vi "CRYSave DataView GUI Info.vi"(11 "DataView Index":i32) -> (3 "DataView GUI Info":T1)   [LabVIEW 2013]
uses:
  Control/Graph Main Info Cluster.ctl
  Control/SplitterBar.ctl
  CRYNew View Global.vi
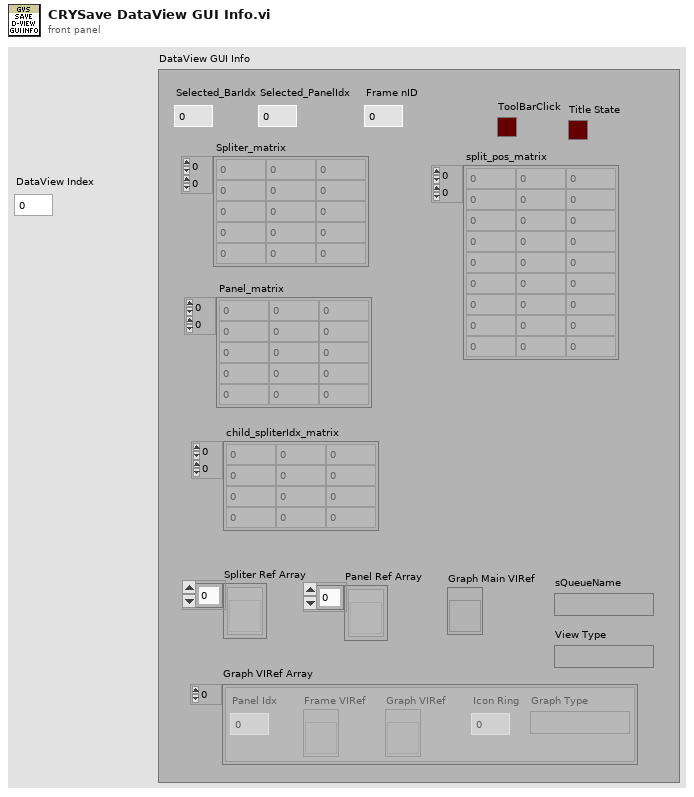
[diagram p1: front panel]
types:
  T1 = typedef "Graph Main Info Cluster.ctl" = cluster{"Selected_BarIdx":i32, "Selected_PanelIdx":i32, "Graph Main VIRef":refnum<vi>, "ToolBarClick":bool, "Spliter Ref Array":refnum<vi>[], "Panel Ref Array":refnum<vi>[], "Spliter_matrix":i32[][], "Panel_matrix":i32[][], "child_spliterIdx_matrix":i32[][], "split_pos_matrix":i32[][], "Title State":bool, "sQueueName":string, "Frame nID":i32, "Graph VIRef Array":cluster{"Graph VIRef":refnum<vi>, "Panel Idx":i32, "Frame VIRef":refnum<vi>, "Icon Ring":i32, "Graph Type":string}[], "View Type":string}
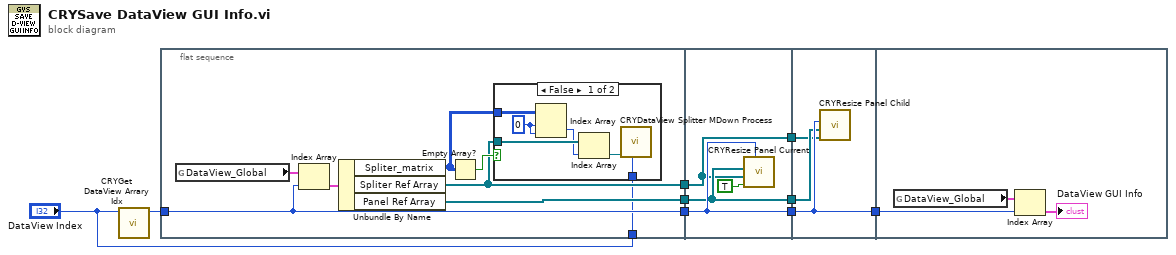
[diagram p0: block diagram]
diagram:
  n1 = call "CRYGet DataView Arrary Idx.vi"("DataView Idx In"="DataView Index") -> ("DataView Arrary Idx out"=w9:i32)  [unwired: 10 in]
  n2 = flat-sequence {
    tunnel: w9 -> [w15]
    tunnel: [w15] -> w8
    tunnel: [w12] -> w7
    tunnel: [w11] -> w6
    tunnel: "DataView Index" -> [w10]
    tunnel: w8 -> [w27]
    tunnel: [w27] -> w5
    tunnel: w7 -> [w25]
    tunnel: w6 -> [w24]
    tunnel: [w25] -> w3
    tunnel: [w24] -> w2
    tunnel: w5 -> [w30]
    tunnel: [w30] -> w4
    tunnel: w3 -> [w29]
    tunnel: w2 -> [w28]
    tunnel: w4 -> [w31]
    frame #0 {
      n3 = global read "CRYNew View Global.vi" "DataView_Global"() -> (w17:T1[])
      n4 = Index Array(array=w17, index=w15) -> (element=w16:T1)
      n5 = Unbundle By Name(w16) -> ("Spliter_matrix"=w14:i32[][], "Spliter Ref Array"=w11:refnum<vi>[], "Panel Ref Array"=w12:refnum<vi>[])
      n6 = Empty Array?(array=w14) -> (empty?=w13:bool)
      n7 = case shown="False" w13 {
        tunnel: w11 -> [w23 _]
        tunnel: w14 -> [w19 _]
        tunnel: w10 -> [w18 _]
        frame False {
          w21 = 0 ("index (row)")
          n8 = Index Array(array=w19, index (row)=w21, index (col)=w21) -> (element=w20:i32)
          n9 = Index Array(array=w23, index=w20) -> (element=w22:refnum<vi>)
          n10 = call "CRYDataView Splitter MDown Process.vi"("DataView Index"=w18, "Selected Spliter Ref"=w22) -> ()  [unwired: 9 in, 1 out]
        }
        frame True {
        }
      }
    }
    frame #1 {
      n11 = call "CRYResize Panel Current.vi"("DataView Array Idx"=w27, "close_panel"=TRUE, "spliter array"=w24, "SubPanel array"=w25) -> ()  [unwired: 8 in]
    }
    frame #2 {
      n12 = call "CRYResize Panel Child.vi"("spliter array"=w28, "SubPanel array"=w29, "DataView Array Idx"=w30) -> ()  [unwired: 9 in]
    }
    frame #3 {
      n13 = global read "CRYNew View Global.vi" "DataView_Global"() -> (w32:T1[])
      n14 = Index Array(array=w32, index=w31) -> (element=→"DataView GUI Info":T1)
    }
  }
